vi "Analog Servo RT.vi"() -> ()   [LabVIEW 2014]
uses:
  <vilib>/userdefined/High Color/nirio_resource_hc.ctl
  <vilib>/FPGAPlugInAG/cRIO-9074/niLvFpga_Open_cRIO-9074.vi
  <vilib>/rvi/interface/common/dynamic/niFpgaDynamicAddResources.vi
  <vilib>/Utility/error.llb/Error Cluster From Error Code.vi
  <vilib>/rvi/errors/niLvFpgaAdjustHostInterfaceError.vi
  <vilib>/FPGAPlugInAG/Dynamic/niLvFpga_Close_Dynamic.vi
  <vilib>/rvi/interface/nirviOpenFPGA/nirviOpenFPGA.xnode
  FPGA Bitfiles/MotorLabAProject_FPGATarget_AnalogServoFPGAR_paWieZl3474.lvbitx
  <vilib>/rvi/interface/nirviReadWriteControl/nirviReadWriteControl.xnode
  <vilib>/rvi/interface/nirviCloseFPGA/nirviCloseFPGA.xnode
  NiFpgaLv.dll
  <vilib>/rvi/interface/Simulation/niFpgaSimulationCallBeginRW.vi
panel:
  out "Set Point in Counts":dbl
  out "Running":bool
  in  "resource name":T1
  in  "stop":bool
  out "Waveform Chart":cluster{dbl, dbl}(graph)
  in  "Desired Set Point Command (Deg)":dbl(knob) scale=0.0..360.0
  in  "Counts/Rev":dbl
  # "insert encoder counts per revolution here"
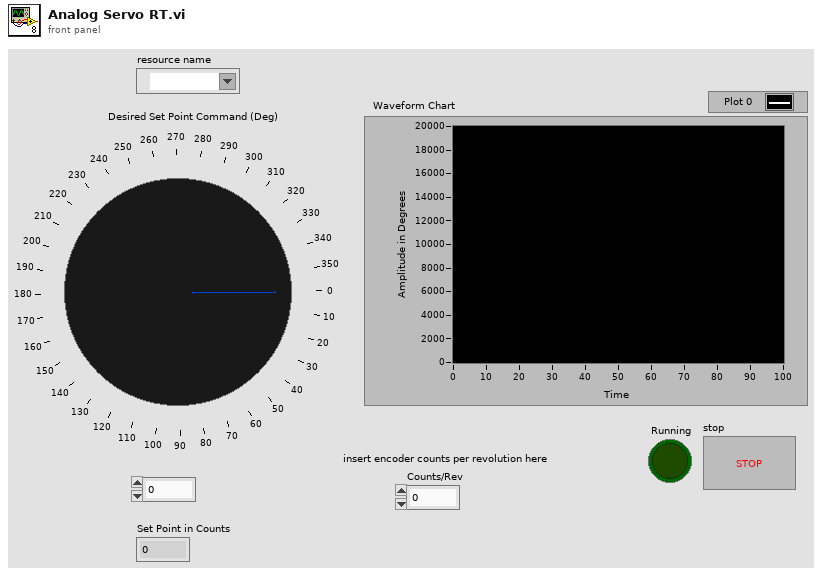
[diagram p1: front panel]
types:
  T1 = typedef "nirio_resource_hc.ctl" = tag
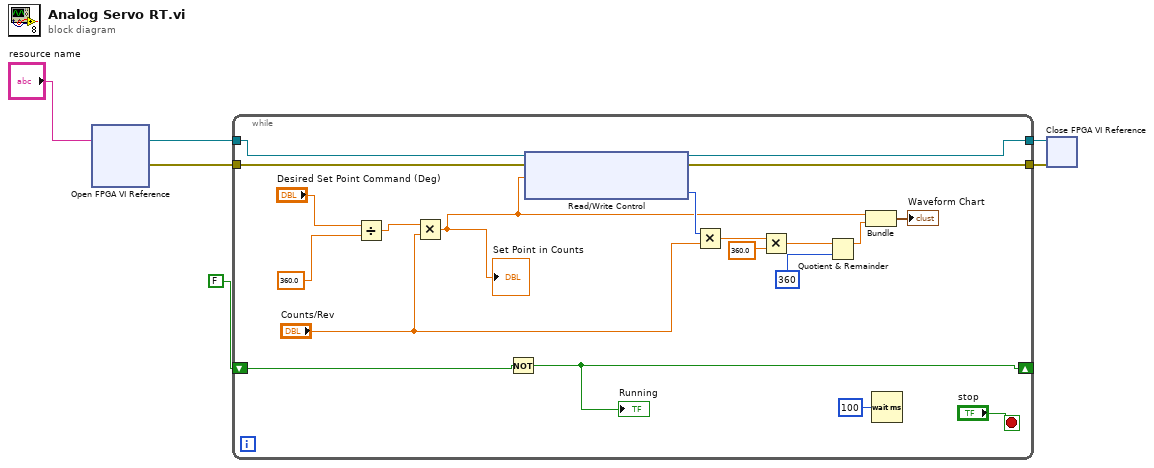
[diagram p0: block diagram]
diagram:
  n1 = xnode "Open FPGA VI Reference"("resource name"="resource name") -> ("FPGA VI Reference Out"=w3:refnum<k20>, "error out"=w6:errorcluster)  [unwired: 1 in]
  n2 = while {
    tunnel: w6 -> [w15]
    tunnel: [w14] -> w5
    tunnel: [w13] -> w4
    tunnel: w3 -> [w12]
    shift-right: [w8] -> _
    shift-left: FALSE -> [w9]
    stop <- "stop" stop-if-true
    n3 = Divide(x="Desired Set Point Command (Deg)", y=360.0) -> (x/y=w19:dbl)
    n4 = Multiply(x=w19, y="Counts/Rev") -> (x*y=w11:dbl)
    "Set Point in Counts" <- w11
    n5 = Not(x=w9) -> (.not. x?=w8:bool)
    "Running" <- w8
    n6 = xnode "Read/Write Control"("FPGA VI Reference In"=w12, "error in"=w15, "Position Command"=w11) -> ("FPGA VI Reference Out"=w14:refnum<k20>, "error out"=w13:errorcluster, "Position Feedback (Counts)"=w24:i32)
    n7 = Multiply(x=w24, y="Counts/Rev") -> (x*y=w26:dbl)
    n8 = Multiply(x=w26, y=360.0) -> (x*y=w23:dbl)
    n9 = Quotient & Remainder(x=w23, y=360) -> (x-y*floor(x/y)=w17:dbl)  [unwired: 1 out]
    n10 = Bundle(w11, w17) -> (→"Waveform Chart":cluster{dbl, dbl})  [unwired: 1 in]
    n11 = Wait (ms)(milliseconds to wait=u32 100) -> ()  [unwired: 1 out]
  }
  n12 = xnode "Close FPGA VI Reference"("FPGA VI Reference In"=w5, "error in"=w4) -> ()  [unwired: 1 out]
